vi "canonLiveview.vi"(9 "Shutter speed":u16(ring) items=["1/8000"=160, "1/6400"=157, "1/6000"=156, "1/5000"=155, "1/4000"=152, "1/3200"=149, "1/3000"=148, "1/2500"=147, "1/2000"=144, "1/1600"=141, "1/1500"=140, "1/1250"=139, "1/100"=136, "1/800"=133, "1/640"=131, "1/500"=128, "1/400"=125, "1/320"=123, "1/250"=120, "1/200"=117, "1/160"=115, "1/125"=112, "1/100"=109, "1/80"=107, "1/60"=104, "1/50"=101, "1/40"=99, "1/30"=96, "1/25"=93, "1/8"=80, "1/6"=77, "1/5"=75, "1/4"=72, "0\"3"=69, "0\"4"=67, "0\"5"=64, "0\"6"=61, "0\"7"=60, "0\"8"=59, "1\""=56, "1\"3"=53, "1\"5"=52, "1\"6"=51, "2\""=48, "2\"5"=45, "3\""=44, "3\"2"=43, "4\""=40, "5\""=37, "6\""=35, "8\""=32, "10\""=29, "13\""=27, "15\""=24, "20\""=21, "25\""=19, "30\""=16], 10 "ISO":u32(ring) items=["Auto"=0, "50"=64, "100"=72, "125"=75, "160"=77, "200"=80, "250"=83, "320"=85, "400"=88, "500"=91, "640"=93, "800"=96, "1000"=99, "1250"=101, "1600"=104, "2000"=107, "2500"=109, "3200"=112, "4000"=115, "5000"=117, "6400"=120, "8000"=123, "10000"=125, "12800"=128, "25600"=136, "51200"=144, "102400"=152, "204800"=160, "409600"=168], 11 "inRef":u32=4294967295) -> (2 "output array":u32[][](array[numeric]), 3 "CamRef":u32)   [LabVIEW 2016]
uses:
  labview for canon om/Vital supporting file for labview program/LV-EDSDK-Distribution_0.2/Distribution/EDSDK-Labview.llb/kEdsProperties.ctl
  labview for canon om/Vital supporting file for labview program/C++/Dll for liveview/x64/Debug/Dll for liveview.dll
panel:
  out "Intensity Graph":dbl[][](graph)
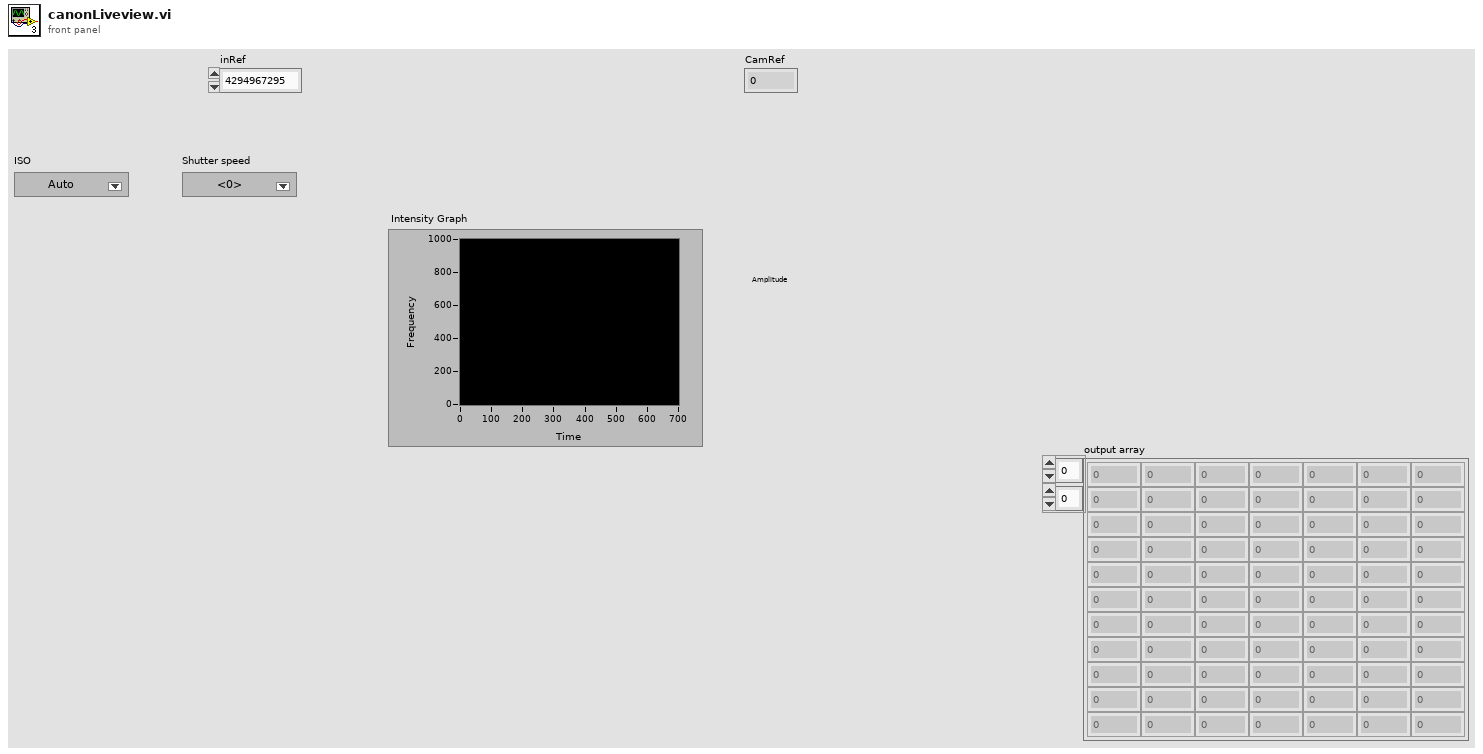
[diagram p1: front panel]
types:
  T1 = typedef "kEdsProperties.ctl" = u32
  T2 = typedef "imagedata.ctl" = cluster{"image type":i32, "image depth":i32, "image":u8[], "mask":u8[], "colors":u32[], "Rectangle":cluster{"left":i16, "top":i16, "right":i16, "bottom":i16}}
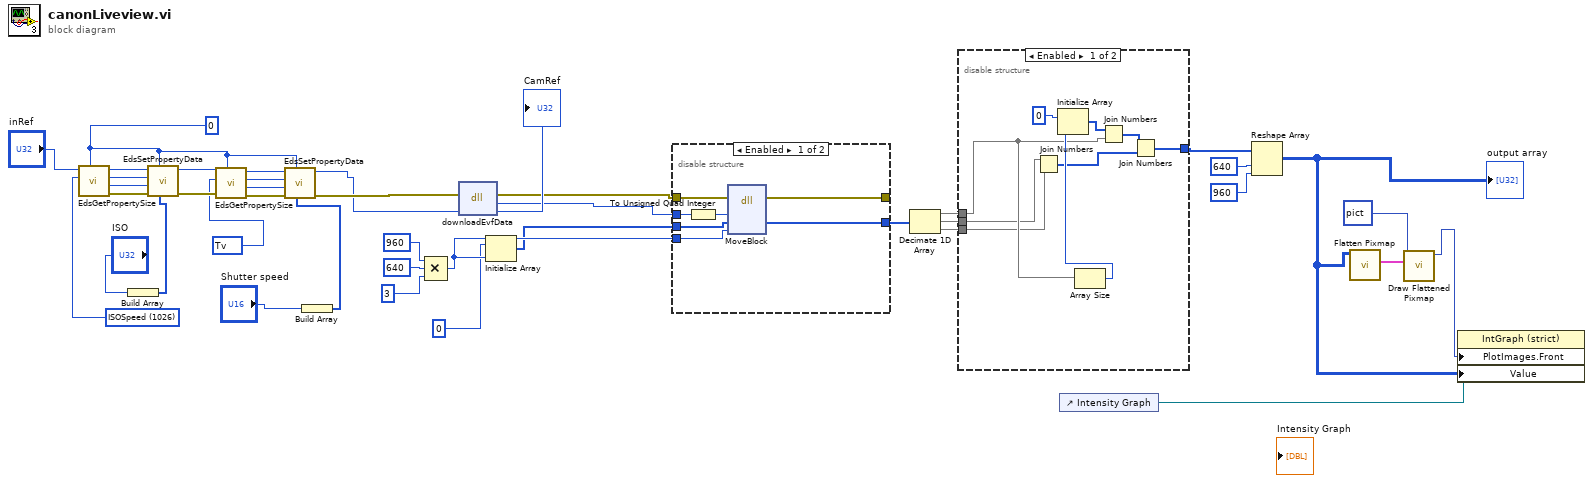
[diagram p0: block diagram]
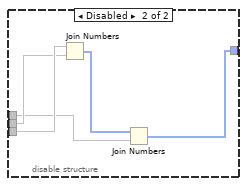
[diagram p2: hidden frame]
diagram:
  w25 = T1 1030 items=["Unknown"=65535, "ProductName"=2, "BodyID"=3, "OwnerName"=4, "MakerName"=5, "DateTime"=6, "FirmwareVersion"=7, "BatteryLevel"=8, "CFn"=9, "SaveTo"=11, "CurrentStorage"=12, "CurrentFolder"=13, "MyMenu"=14, "BatteryQuality"=16, "HDDirectoryStructure"=32, "ImageQuality"=256, "JpegQuality"=257, "Orientation"=258, "ICCProfile"=259, "FocusInfo"=260, "DigitalExposure"=261, "WhiteBalance"=262, "ColorTemperature"=263, "WhiteBalanceShift"=264, "Contrast"=265, "ColorSaturation"=266, "ColorTone"=267, "Sharpness"=268, "ColorSpace"=269, "ToneCurve"=270, "PhotoEffect"=271, "FilterEffect"=272, "ToningEffect"=273, "ParameterSet"=274, "ColorMatrix"=275, "PictureStyle"=276, "PictureStyleDesc"=277, "ETTL2Mode"=279, "PictureStyleCaption"=512, "Linear"=768, "ClickWBPoint"=769, "WBCoeffs"=770, "GPSVersionID"=2048, "GPSLatitudeRef"=2049, "GPSLatitude"=2050, "GPSLongitudeRef"=2051, "GPSLongitude"=2052, "GPSAltitudeRef"=2053, "GPSAltitude"=2054, "GPSTimeStamp"=2055, "GPSSatellites"=2056, "GPSStatus"=2057, "GPSMapDatum"=2066, "GPSDateStamp"=2077, "AtCapture_Flag"=2147483648, "AEMode"=1024, "DriveMode"=1025, "ISOSpeed"=1026, "MeteringMode"=1027, "AFMode"=1028, "Av"=1029, "Tv"=1030, "ExposureCompensation"=1031, "FlashCompensation"=1032, "FocalLength"=1033, "AvailableShots"=1034, "Bracket"=1035, "WhiteBalanceBracket"=1036, "LensName"=1037, "AEBracket"=1038, "FEBracket"=1039, "ISOBracket"=1040, "NoiseReduction"=1041, "FlashOn"=1042, "RedEye"=1043, "FlashMode"=1044, "LensStatus"=1046, "Artist"=1048, "Copyright"=1049, "DepthOfField"=1051, "EFCompensation"=1054, "Evf_OutputDevice"=1280, "Evf_Mode"=1281, "Evf_WhiteBalance"=1282, "Evf_ColorTemperature"=1283, "Evf_DepthOfFieldPreview"=1284, "Evf_Zoom"=1287, "Evf_ZoomPosition"=1288, "Evf_FocusAid"=1289, "Evf_Histogram"=1290, "Evf_ImagePosition"=1291, "Evf_HistogramStatus"=1292, "Evf_AFMode"=1294, "Evf_CoordinateSystem"=1344, "Evf_ZoomRect"=1345] ("inPropertyID")
  w27 = 0 ("inParam")
  w37 = T1 1026 items=["Unknown"=65535, "ProductName"=2, "BodyID"=3, "OwnerName"=4, "MakerName"=5, "DateTime"=6, "FirmwareVersion"=7, "BatteryLevel"=8, "CFn"=9, "SaveTo"=11, "CurrentStorage"=12, "CurrentFolder"=13, "MyMenu"=14, "BatteryQuality"=16, "HDDirectoryStructure"=32, "ImageQuality"=256, "JpegQuality"=257, "Orientation"=258, "ICCProfile"=259, "FocusInfo"=260, "DigitalExposure"=261, "WhiteBalance"=262, "ColorTemperature"=263, "WhiteBalanceShift"=264, "Contrast"=265, "ColorSaturation"=266, "ColorTone"=267, "Sharpness"=268, "ColorSpace"=269, "ToneCurve"=270, "PhotoEffect"=271, "FilterEffect"=272, "ToningEffect"=273, "ParameterSet"=274, "ColorMatrix"=275, "PictureStyle"=276, "PictureStyleDesc"=277, "ETTL2Mode"=279, "PictureStyleCaption"=512, "Linear"=768, "ClickWBPoint"=769, "WBCoeffs"=770, "GPSVersionID"=2048, "GPSLatitudeRef"=2049, "GPSLatitude"=2050, "GPSLongitudeRef"=2051, "GPSLongitude"=2052, "GPSAltitudeRef"=2053, "GPSAltitude"=2054, "GPSTimeStamp"=2055, "GPSSatellites"=2056, "GPSStatus"=2057, "GPSMapDatum"=2066, "GPSDateStamp"=2077, "AtCapture_Flag"=2147483648, "AEMode"=1024, "DriveMode"=1025, "ISOSpeed"=1026, "MeteringMode"=1027, "AFMode"=1028, "Av"=1029, "Tv"=1030, "ExposureCompensation"=1031, "FlashCompensation"=1032, "FocalLength"=1033, "AvailableShots"=1034, "Bracket"=1035, "WhiteBalanceBracket"=1036, "LensName"=1037, "AEBracket"=1038, "FEBracket"=1039, "ISOBracket"=1040, "NoiseReduction"=1041, "FlashOn"=1042, "RedEye"=1043, "FlashMode"=1044, "LensStatus"=1046, "Artist"=1048, "Copyright"=1049, "DepthOfField"=1051, "EFCompensation"=1054, "Evf_OutputDevice"=1280, "Evf_Mode"=1281, "Evf_WhiteBalance"=1282, "Evf_ColorTemperature"=1283, "Evf_DepthOfFieldPreview"=1284, "Evf_Zoom"=1287, "Evf_ZoomPosition"=1288, "Evf_FocusAid"=1289, "Evf_Histogram"=1290, "Evf_ImagePosition"=1291, "Evf_HistogramStatus"=1292, "Evf_AFMode"=1294, "Evf_CoordinateSystem"=1344, "Evf_ZoomRect"=1345] ("inPropertyID")
  n1 = call "EdsGetPropertySize.vi"("inParam"=w27, "inPropertyID"=w37, "inRef"="inRef") -> ("error out"=w39:errorcluster, "outSize"=w38:u32, "inPropertyID dup"=w40:T1, "inRef dup"=w41:u32)  [unwired: 4 in, 1 out]
  n2 = Build Array("ISO") -> (w35:u32[])
  n3 = call "EdsSetPropertyData.vi"("inPropertyData"=w35, "inParam"=w27, "error in"=w39, "inPropertySize"=w38, "inPropertyID"=w40, "inRef"=w41) -> ("error out"=w33:errorcluster, "inRef dup"=w26:u32)  [unwired: 4 in]
  n4 = call "EdsGetPropertySize.vi"("inParam"=w27, "error in"=w33, "inPropertyID"=w25, "inRef"=w26) -> ("error out"=w32:errorcluster, "outSize"=w30:u32, "inPropertyID dup"=w34:T1, "inRef dup"=w31:u32)  [unwired: 3 in, 1 out]
  n5 = Build Array("Shutter speed") -> (w28:u16[])
  n6 = call "EdsSetPropertyData.vi"("inPropertyData"=w28, "inParam"=w27, "error in"=w32, "inPropertySize"=w30, "inPropertyID"=w34, "inRef"=w31) -> ("error out"=w24:errorcluster, "inRef dup"=w23:u32)  [unwired: 4 in]
  n7 = Compound Arithmetic op=MULTIPLY(960 ("dimension size"), 640 ("dimension size"), 3 ("dimension size")) -> (w19:i32)
  n8 = dll-call lib="D:/All users/PoSheng/src/labview for canon om/Vital supporting file for labview program/C++/Dll for liveview/x64/Debug/Dll for liveview.dll" fn="downloadEvfData"(error in=w24, "CamRef"=w23) -> (error out=w13:errorcluster, "return type"=w12:i64, "CamRef"=→"CamRef":u32)  [unwired: 2 in, 1 out]
  n9 = Initialize Array ("初始化数组")(u8 0 ("element"), w19) -> (w18:u8[])
  n10 = disable-structure shown="Enabled" {
    disable-tunnel: [w48 w49] -> _
    disable-tunnel: w12 -> [w47 _]
    disable-tunnel: w13 -> [w46 w49]
    disable-tunnel: w18 -> [w45 _]
    disable-tunnel: w19 -> [w44 _]
    disable-tunnel: [w42 _] -> w20
    frame Enabled {
      n11 = To Unsigned Quad Integer(1:w47) -> (0:w43:u64)
      n12 = dll-call lib="LabVIEW" fn="MoveBlock"(error in=w46, "src"=w43, "dst"=w45, "size"=w44) -> (error out=w48:errorcluster, "dst"=w42:u8[])  [unwired: 5 in, 1 out]
    }
    frame Disabled {
    }
  }
  n13 = Decimate 1D Array(w20) -> (w11:u8[], w10:u8[], w9:u8[])
  n14 = disable-structure shown="Enabled" {
    disable-tunnel: w10 -> [w51 w60]
    disable-tunnel: w11 -> [w52 w59]
    disable-tunnel: w9 -> [w50 w61]
    disable-tunnel: [w53 w62] -> w2
    frame Enabled {
      n15 = Join Numbers(hi=w51, lo=w50) -> ((hi.lo)=w54:u16[])
      n16 = Array Size(array=w52) -> (size(s)=w57:i32)
      n17 = Initialize Array(u8 0, w57) -> (w56:u8[])
      n18 = Join Numbers(hi=w56, lo=w52) -> ((hi.lo)=w55:u16[])
      n19 = Join Numbers(hi=w55, lo=w54) -> ((hi.lo)=w53:u32[])
    }
    frame Disabled {
      n20 = Join Numbers(hi=w61, lo=w60) -> ((hi.lo)=w63:u16[])
      n21 = Join Numbers(hi=w63, lo=w59) -> ((hi.lo)=w62:u32[])
    }
  }
  n22 = control-ref of="Intensity Graph"() -> (w1:refnum<vi>)
  n23 = Reshape Array(w2, 640 ("dimension size"), 960 ("dimension size")) -> (w3:u32[][])
  "output array" <- w3
  n24 = call <vilib>:"Flatten Pixmap.vi"("24-bit pixmap"=w3) -> ("image data"=w8:T2)  [unwired: 10 in]
  n25 = call <vilib>:"Draw Flattened Pixmap.vi"("image data"=w8, "picture"=picture data[5B]) -> ("new picture"=w5:picture)  [unwired: 7 in]
  n26 = property on="Property Node" class="IntGraph (strict)"(reference=w1, "PlotImages.Front"=w5, "Value"=w3) -> ()  [unwired: 1 in, 2 out]
